vi "Variable@LFindIndexSet__Parameter.vi"(1 "ParamterIn":string) -> (0 "ParamterOut":string)   [LabVIEW 2019]
panel:
  in  "Value":string(combo)
  in  "Section":string(combo)
  in  "VarS":string(combo)
  in  "ParameterName":string(combo)
  in  "Confirm":bool
  # "Variable@LFindIndexSet $Variable,$Value,Var1(,Var2,.....,$Section)"
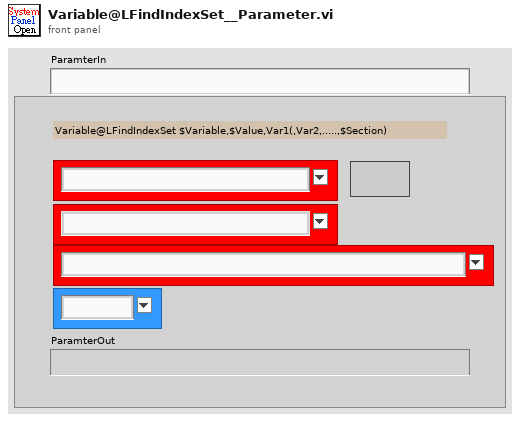
[diagram p1: front panel]
types:
  T1 = enum16{"Get", "Init", "Set", "Delete", "GetElement", "Inc", "Dec", "ReName"}
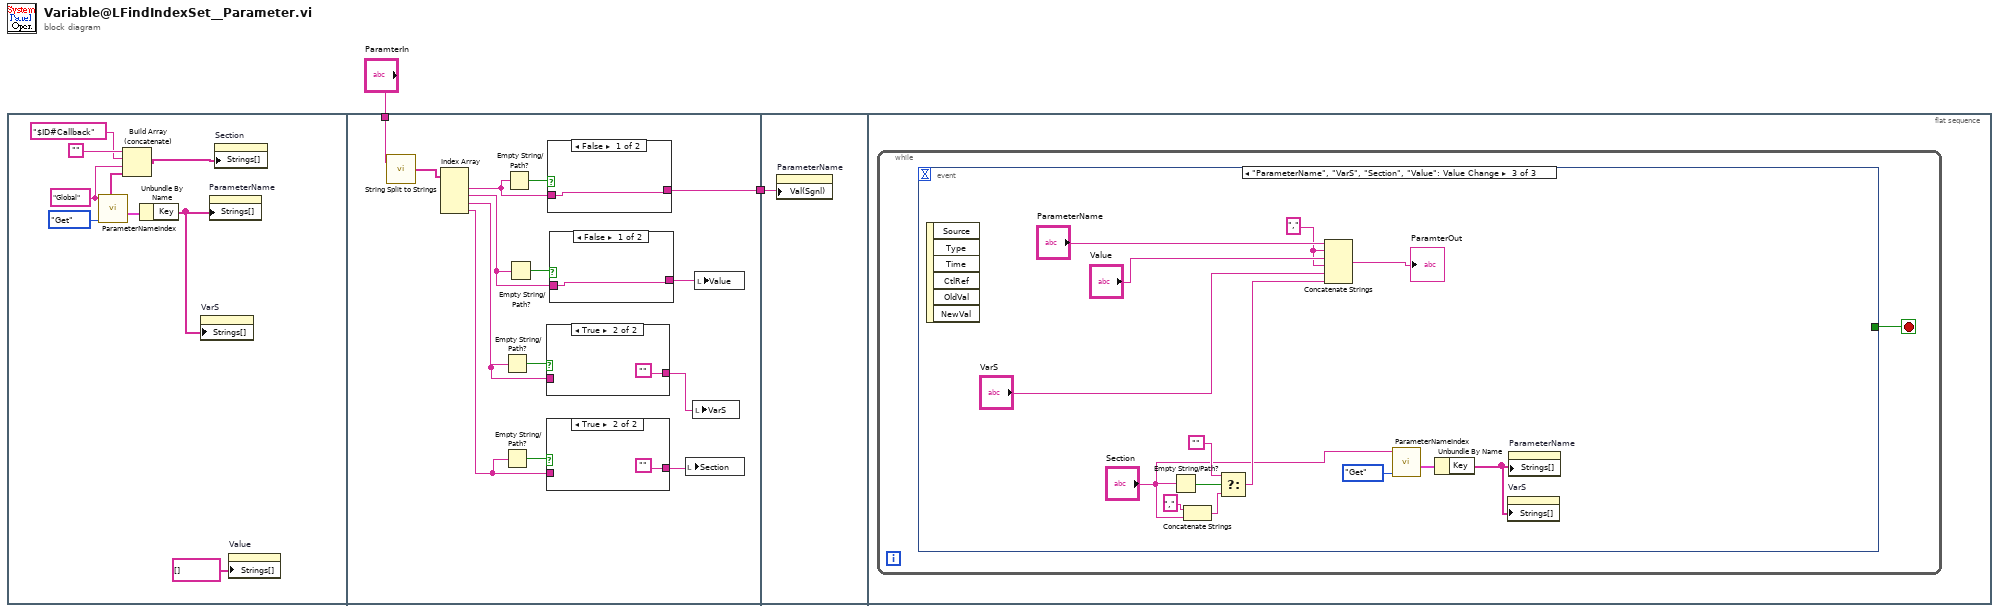
[diagram p0: block diagram]
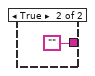
[diagram p2: hidden frame]
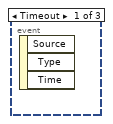
[diagram p6: hidden frame]
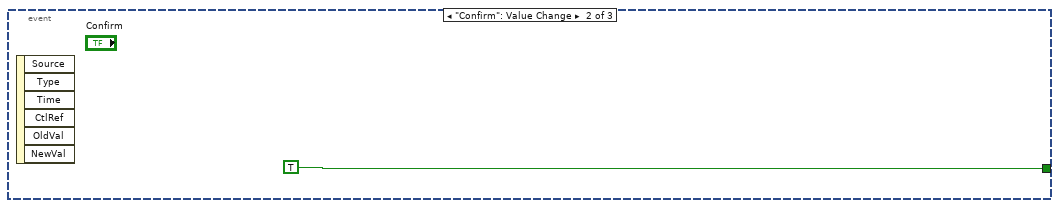
[diagram p7: hidden frame]
diagram:
  n1 = flat-sequence {
    tunnel: "ParamterIn" -> [w21]
    tunnel: [w23] -> w1
    tunnel: w1 -> [w34]
    frame #0 {
      w4 = "Global" ("VariableSection")
      n2 = call "ParameterNameIndex.vi"("OP"=T1."Get", "VariableSection"=w4) -> ("GlobalKeyValue"=w11:cluster{"Key":string[], "Value":string[]}, "SectionList"=w7:string[])  [unwired: 3 in, 5 out]
      n3 = Build Array (concatenate)("", "$ID#Callback" ("VariableSection"), w4, w7) -> (w6:string[])
      n4 = Unbundle By Name(w11) -> ("Key"=w8:string[])
      n5 = property on="VarS" class="CmbBox"("Strings[]"=w8) -> ()  [unwired: 2 in, 2 out]
      n6 = property on="ParameterName" class="CmbBox"("Strings[]"=w8) -> ()  [unwired: 2 in, 2 out]
      n7 = property on="Section" class="CmbBox"("Strings[]"=w6) -> ()  [unwired: 2 in, 2 out]
      n8 = property on="Value" class="CmbBox"("Strings[]"=string[] [] ("Strings []")) -> ()  [unwired: 2 in, 2 out]
    }
    frame #1 {
      n9 = call "String Split to Strings.vi"("String"=w21) -> ("Array"=w20:string[])  [unwired: 1 in]
      n10 = Index Array(array=w20) -> (element #1=w19:string, element #2=w13:string, element #3=w15:string, element #4=w16:string)  [unwired: 4 in]
      n11 = Empty String/Path?(string/path=w15) -> (empty?=w24:bool)
      n12 = Empty String/Path?(string/path=w16) -> (empty?=w18:bool)
      n13 = Empty String/Path?(string/path=w19) -> (empty?=w25:bool)
      n14 = Empty String/Path?(string/path=w13) -> (empty?=w14:bool)
      n15 = case shown="True" w24 {
        tunnel: w15 -> [w30 _]
        tunnel: [w30 ""] -> w22
        frame False {
        }
        frame True {
        }
      }
      n16 = case shown="True" w18 {
        tunnel: w16 -> [w28 _]
        tunnel: [w28 ""] -> w17
        frame False {
        }
        frame True {
        }
      }
      n17 = case shown="False" w25 {
        tunnel: w19 -> [w32 w33]
        tunnel: [w32 w33] -> w23
        frame False {
        }
        frame True {
        }
      }
      n18 = case shown="False" w14 {
        tunnel: w13 -> [w26 _]
        tunnel: [w26 ""] -> w12
        frame False {
        }
        frame True {
        }
      }
      n19 = local write "Section"(w17) -> ()
      n20 = local write "VarS"(w22) -> ()
      n21 = local write "Value"(w12) -> ()
    }
    frame #2 {
      n22 = property on="ParameterName" class="CmbBox"("Val(Sgnl)"=w34) -> ()  [unwired: 2 in, 2 out]
    }
    frame #3 {
      n23 = while {
        stop <- w35 stop-if-true
        n24 = event shown="[2] \"ParameterName\", \"VarS\", \"Section\", \"Value\": Value Change" {
          selector: _ -> [_ _ _]
          dyn-events: _ -> [_ _ _]
          timeout: _ -> [_ _ _]
          tunnel: [_ TRUE _] -> w35
          event Timeout {
            n25 = event-data() -> ()  [unwired: 1 in, 3 out]
          }
          event "Confirm": Value Change {
            n26 = event-data() -> ()  [unwired: 1 in, 6 out]
          }
          event "ParameterName", "VarS", "Section", "Value": Value Change {
            w43 = "," ("string")
            n27 = event-data() -> ()  [unwired: 1 in, 6 out]
            n28 = Empty String/Path?(string/path="Section") -> (empty?=w46:bool)
            n29 = Concatenate Strings("," ("string"), "Section") -> (w47:string)
            n30 = Select(t="", s=w46, f=w47) -> (s? t:f=w41:string)
            n31 = Concatenate Strings("ParameterName", w43, "Value", w43, "VarS", w41) -> (→"ParamterOut":string)
            n32 = call "ParameterNameIndex.vi"("OP"=T1."Get", "VariableSection"="Section") -> ("GlobalKeyValue"=w38:cluster{"Key":string[], "Value":string[]})  [unwired: 3 in, 6 out]
            n33 = Unbundle By Name(w38) -> ("Key"=w40:string[])
            n34 = property on="VarS" class="CmbBox"("Strings[]"=w40) -> ()  [unwired: 2 in, 2 out]
            n35 = property on="ParameterName" class="CmbBox"("Strings[]"=w40) -> ()  [unwired: 2 in, 2 out]
          }
        }
      }
    }
  }
